vi "Pressure_Monitor_bkfl.vi"(11 "VISA resource name":refnum<visa-resource-name>) -> (0 "Error at segmenting output":errorcluster, 1 "Error at VISA Read":errorcluster, 3 "Flow readout":dbl)   [LabVIEW 2015]
uses:
  <vilib>/Utility/config.llb/Read Key (I32).vi
  <vilib>/Utility/config.llb/NI_LVConfig.lvlib
panel:
  out "concatenated string":string
  out "Waveform Chart 2":dbl(graph)
  out "date/time string 2":string
  out "current time 2":timestamp
  out "decimal integer string":string
  out "remaining string":string
  out "read buffer":string
  out "result":bool
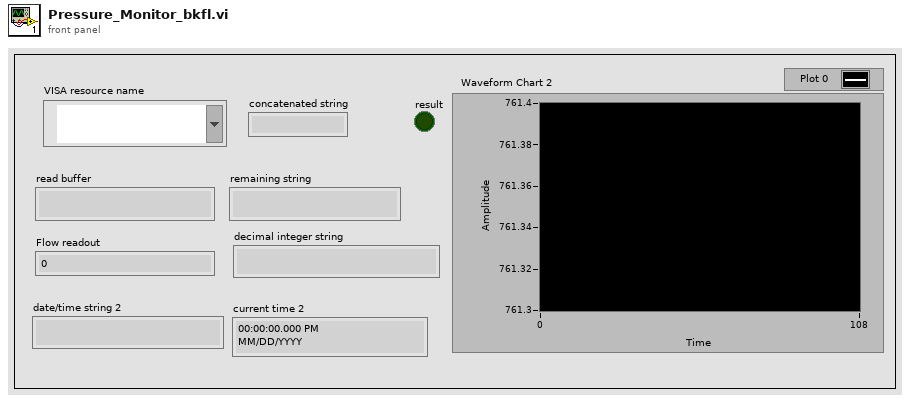
[diagram p1: front panel]
types:
  T1 = typedef "NI_LVConfig.lvlib/Config Data RefNum.ctl" = refnum<k1>
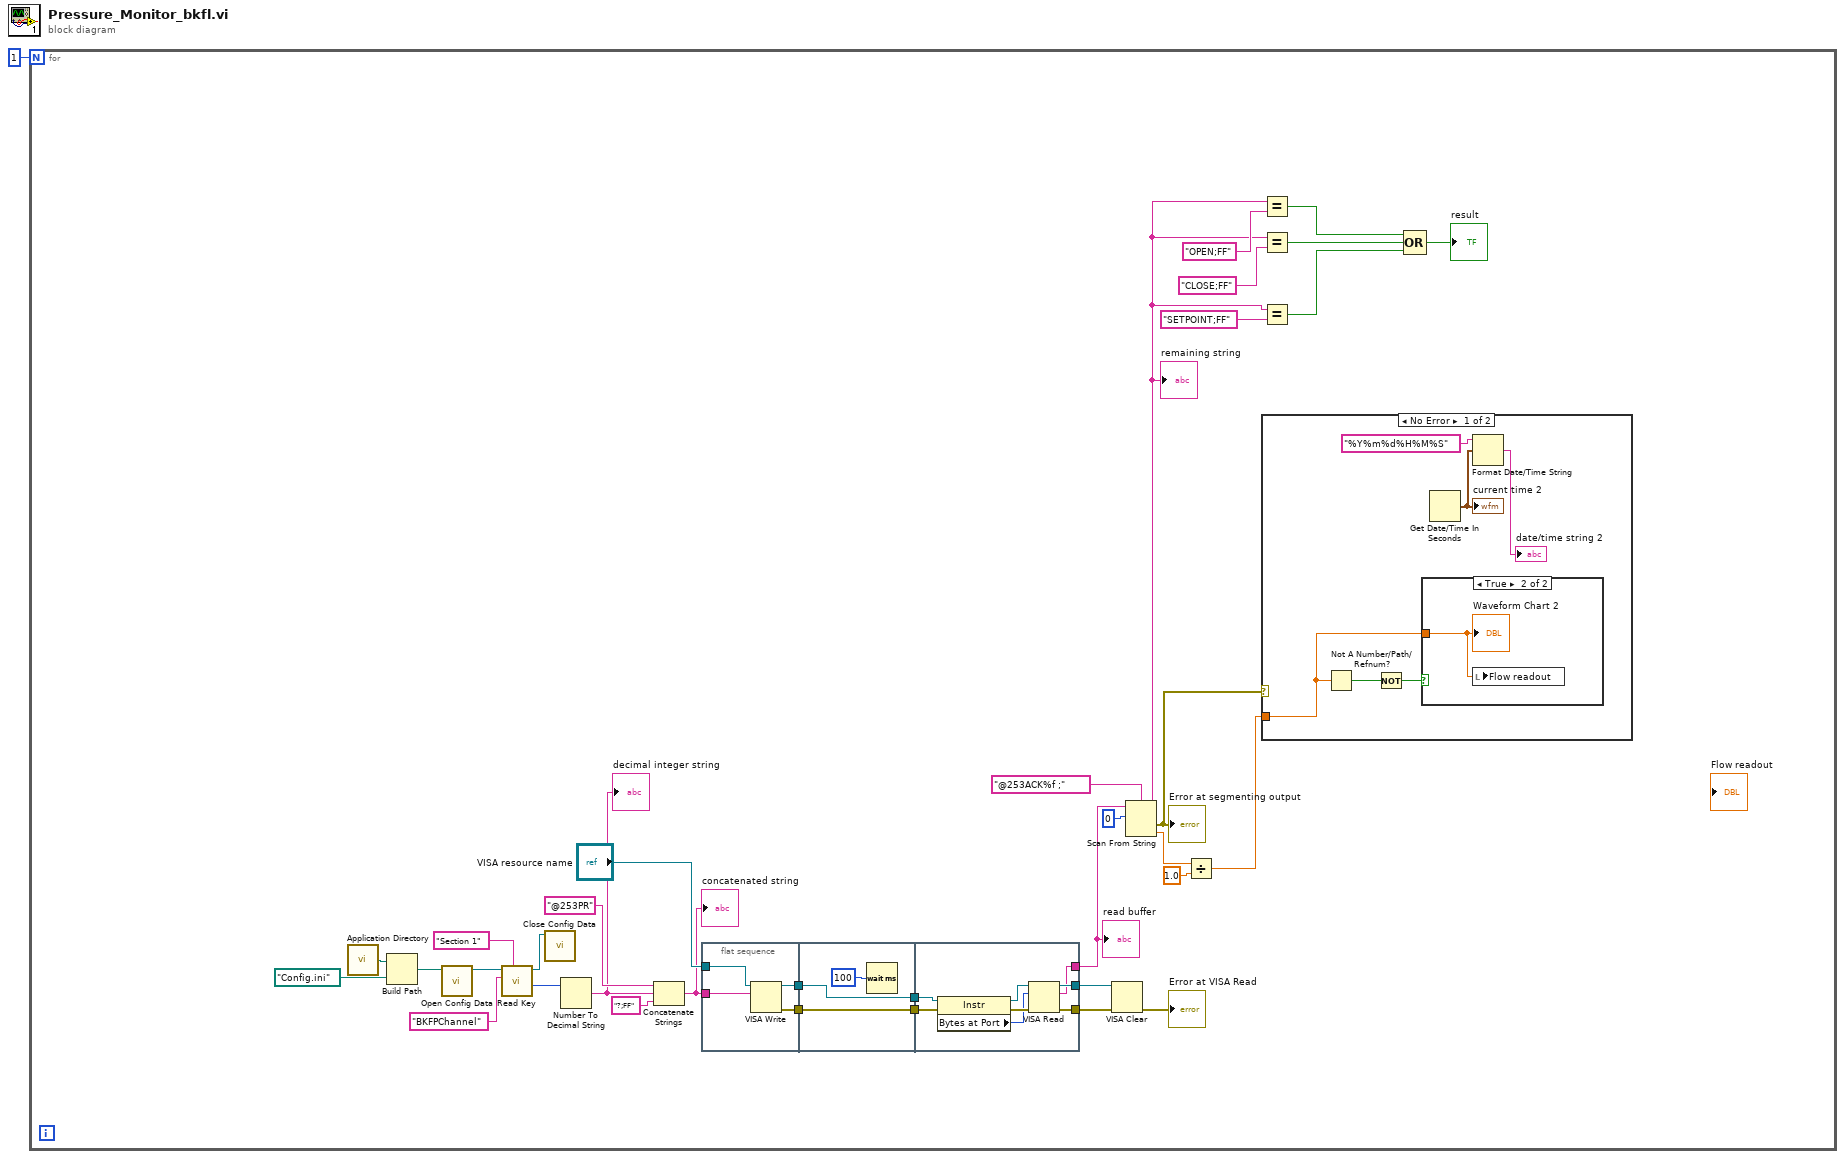
[diagram p0: block diagram]
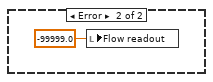
[diagram p3: hidden frame]
diagram:
  n1 = for {
    N: 1 -> [_]
    n2 = call <vilib>:"Application Directory.vi"() -> ("Application Directory"=w17:path)
    n3 = Build Path(base path=w17, name or relative path=path "Config.ini" ("default name")) -> (appended path=w21:path)
    n4 = call <vilib>:"Open Config Data.vi"("configuration file path"=w21) -> ("refnum"=w28:T1)  [unwired: 8 in, 2 out]
    n5 = call-poly <vilib>:"Read Key.vi"("section"="Section 1", "key"="BKFPChannel", "refnum"=w28) -> ("value"=w25:i32, "refnum out"=w26:T1)  [unwired: 5 in, 2 out]
    n6 = call <vilib>:"Close Config Data.vi"("refnum"=w26) -> ()  [unwired: 9 in, 2 out]
    n7 = Number To Decimal String(number=w25) -> (decimal integer string=w23:string)  [unwired: 1 in]
    "decimal integer string" <- w23
    n8 = Concatenate Strings("@253PR" ("string"), w23, "?;FF" ("string")) -> (w5:string)
    "concatenated string" <- w5
    n9 = flat-sequence {
      tunnel: w5 -> [w40]
      tunnel: "VISA resource name" -> [w39]
      tunnel: [w38] -> w36
      tunnel: [w37] -> w35
      tunnel: w36 -> [w42]
      tunnel: [w42] -> w34
      tunnel: w35 -> [w41]
      tunnel: [w41] -> w33
      tunnel: w34 -> [w48]
      tunnel: w33 -> [w47]
      tunnel: [w46] -> w4
      tunnel: [w45] -> w3
      tunnel: [w44] -> w2
      frame #0 {
        n10 = VISA Write(VISA resource name=w39, write buffer=w40) -> (VISA resource name out=w38:refnum<visa-resource-name>, error out=w37:errorcluster)  [unwired: 1 in, 1 out]
      }
      frame #1 {
        n11 = Wait (ms)(milliseconds to wait=u32 100) -> ()  [unwired: 1 out]
      }
      frame #2 {
        n12 = property class="Instr"(reference=w48, error in=w47) -> (reference out=w49:refnum<visa-resource-name>, error out=w51:errorcluster, "Bytes at Port"=w50:u32)
        n13 = VISA Read(VISA resource name=w49, byte count=w50, error in (no error)=w51) -> (VISA resource name out=w46:refnum<visa-resource-name>, read buffer=w44:string, error out=w45:errorcluster)  [unwired: 1 out]
      }
    }
    n14 = VISA Clear(VISA resource name=w4, error in (no error)=w3) -> (error out=→"Error at VISA Read":errorcluster)  [unwired: 1 out]
    n15 = Scan From String(format string="@253ACK%f ;", input string=w2, initial scan location=u32 0) -> (remaining string=w10:string, error out=w8:errorcluster, output 1=w19:dbl)  [unwired: 2 in, 1 out]
    "Error at segmenting output" <- w8
    "remaining string" <- w10
    n16 = Divide(x=w19, y=1.0) -> (x/y=w18:dbl)
    n17 = Equal?(x=w10, y="OPEN;FF") -> (x = y?=w15:bool)
    n18 = Equal?(x=w10, y="CLOSE;FF") -> (x = y?=w14:bool)
    n19 = Equal?(x=w10, y="SETPOINT;FF") -> (x = y?=w11:bool)
    n20 = case shown="No Error" w8 {
      tunnel: w18 -> [w53 _]
      frame No Error {
        n21 = Not A Number/Path/Refnum?(number/path/refnum=w53) -> (NaN/Path/Refnum?=w55:bool)
        n22 = Not(x=w55) -> (.not. x?=w54:bool)
        n23 = case shown="True" w54 {
          tunnel: w53 -> [_ w58]
          frame False {
          }
          frame True {
            n24 = local write "Flow readout"(w58) -> ()
            "Waveform Chart 2" <- w58
          }
        }
        n25 = Get Date/Time In Seconds() -> (seconds since 1Jan1904=w57:timestamp)
        "current time 2" <- w57
        n26 = Format Date/Time String(time format string (%c)="%Y%m%d%H%M%S", seconds (now)=w57) -> (date/time string=→"date/time string 2":string)  [unwired: 1 in]
      }
      frame Error {
        n27 = local write "Flow readout"(-99999.0) -> ()
      }
    }
    n28 = Compound Arithmetic op=OR(w15, w14, w11) -> (→"result":bool)
    "read buffer" <- w2
  }
